vi "Set Window Icon.vi"(7 "Icon Type":enum32{"Small", "Big"}(ring), 8 "error in (no error)":errorcluster, 10 "VIRef (calling VI)":refnum<vi>, 11 "RGB Image":u32[][](array[numeric])) -> (0 "Error Out":errorcluster)   [LabVIEW 2023, in "Font Glyph Drawer Interface.lvlib" / "VI Icon Canvas.lvclass"]
doc: "Set a custom title bar icon for the referenced VI.\nIf no VI reference is supplied the VI calling this function is altered.\n\nUse <b>set</b> to change the icon to a custom icon, and <b>reset</b> to revert the icon to the previous value."
uses:
  VI Icon Canvas.lvclass
  VI Icon Canvas.lvclass/VI Icon Canvas.ctl
  user32.dll
  gdi32.dll
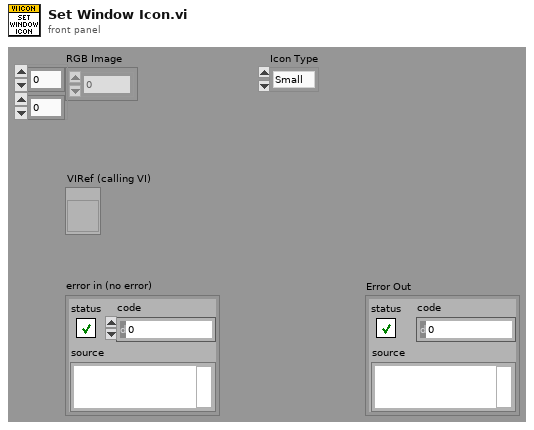
[diagram p1: front panel]
types:
  T1 = cluster{"fIcon":i32, "xHotspot":u32, "yHotspot":u32, "hbmMask":u32, "hbmColor":u32}
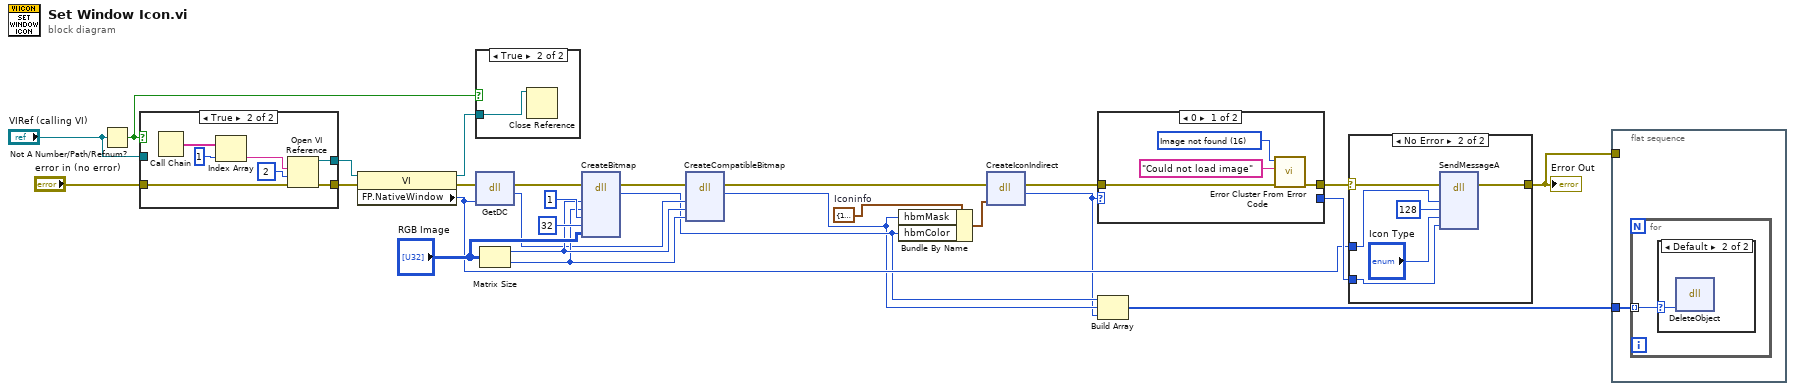
[diagram p0: block diagram]
diagram:
  w15 = T1 {"fIcon"=1, "xHotspot"=0, "yHotspot"=0, "hbmMask"=0, "hbmColor"=0}  # Iconinfo
  n1 = Not A Number/Path/Refnum?(number/path/refnum="VIRef (calling VI)") -> (NaN/Path/Refnum?=w22:bool)
  n2 = case shown="True" w22 {
    tunnel: [w29 w36] -> w26
    tunnel: "VIRef (calling VI)" -> [w29 _]
    tunnel: "error in (no error)" -> [w28 w31]
    tunnel: [w28 w30] -> w1
    frame False {
    }
    frame True {
      n3 = Call Chain() -> (call chain=w32:string[])
      n4 = Index Array(array=w32, index=1 ("Index")) -> (element=w34:string)
      n5 = Open VI Reference(vi path=w34, options=2, error in (no error)=w31) -> (vi reference=w36:refnum<vi>, error out=w30:errorcluster)  [unwired: 3 in]
    }
  }
  n6 = property class="VI"(reference=w26, error in=w1) -> (reference out=w23:refnum<vi>, error out=w12:errorcluster, "FP.NativeWindow"=w8:u64)
  n7 = case shown="True" w22 {
    tunnel: w23 -> [_ w37]
    frame False {
    }
    frame True {
      n8 = Close Reference(reference=w37) -> ()  [unwired: 1 in, 1 out]
    }
  }
  n9 = dll-call lib="user32.dll" fn="GetDC"(error in=w12, "HWND"=w8) -> (error out=w11:errorcluster, "HDC"=w13:u32)  [unwired: 3 in, 1 out]
  n10 = Matrix Size(0:"RGB Image") -> (1:w17:i32, 2:w16:i32)
  n11 = dll-call lib="gdi32.dll" fn="CreateBitmap"(error in=w11, "nWidth"=w17, "nHeight"=w16, "nPlanes"=u32 1, "nBitCount"=u32 32, "lpBits"="RGB Image") -> (error out=w18:errorcluster, "HBITMAP"=w7:u32)  [unwired: 7 in, 1 out]
  n12 = dll-call lib="gdi32.dll" fn="CreateCompatibleBitmap"(error in=w18, "hdc"=w13, "cx"=w17, "cy"=w16) -> (error out=w14:errorcluster, "HICON"=w6:u32)  [unwired: 5 in, 1 out]
  n13 = Bundle By Name(cluster=w15, "hbmMask"=w6, "hbmColor"=w7) -> (w10:T1)
  n14 = dll-call lib="user32.dll" fn="CreateIconIndirect"(error in=w14, "piconinfo"=w10) -> (error out=w9:errorcluster, "HICON"=w5:u32)  [unwired: 3 in, 1 out]
  n15 = case shown="0" w5 {
    selector: w5 -> [_ w42]
    tunnel: [_ w42] -> w24
    tunnel: [w39 w43] -> w25
    tunnel: w9 -> [w38 w43]
    frame 0 {
      w41 = 16 items=["No error", "Argument error", "Memory is full", "Out of zone", "End of file", "File already open", "Generic file I/O error", "File not found", "File permission error", "Disk is full", "Duplicate path", "Too many files open", "System feature not enabled", "Resource file not found", "Cannot add resource", "Resource not found", "Image not found", "Image memory error", "Pen does not exist", "Config type invalid", "Config token not found", "Config parse error", "Config memory error", "Bad external code format", "Bad external code offset", "External code not present", "Null window", "Destroy window error", "Null menu", "Print aborted", "Bad print record", "Print driver error", "Windows error during printing", "Memory error during printing", "Print dialog error", "Generic print error", "Invalid device refnum", "Device not found", "Device parameter error", "Device unit error", "Cannot open device", "Device call aborted", "Generic error", "Cancelled by user", "Object ID too low", "Object ID too high", "Object not in heap", "Unknown heap", "Unknown object (invalid DefProc)", "Unknown object (DefProc not in table)", "Message out of range", "Invalid (null) method", "Unknown message", "Manager call not supported", "Bad address", "Network operation in progress", "Network operation timed out", "Connection is busy", "Network attribute not supported", "Network error", "Address in use", "System out of memory", "Connection aborted", "Connection refused", "Not connected", "Already connected", "Connection closed", "Initialization error (interapplication manager)", "Bad occurrence", "Wait on unbound occurrence handler", "Occurrence queue overflow", "Datalog type conflict", "Unused", "Unrecognized type (interapplication manager)", "Memory corrupt", "Failed to make temporary DLL", "Old CIN version", "Drag socket not found", "Failed to load drop-object", "Failed to register OLE object", "Failed to release OLE object", "Format specifier type mismatch", "Unknown format specifier", "Too few format specifiers", "Too many format specifiers", "Scan failed", "Newer CIN version", "Error converting to variant", "Runtime menu error", "Password tampered", "Variant attribute not found", "Incompatible variant data type", "Event data is not available", "Event Store is not present", "Occurrence is not found", "Event Queue is not created", "Event info is not available", "Refnum passed is NULL", "Error retrieving Class GUID", "Error retrieving CoClass GUID", "Error retrieving TypeLib GUID.", "Bad built application magic bytes.", "Specific driver is different from the specific driver associated with the Logical Name.", "There is no session opened to the class driver.", "Max Error", "MAX - Error with config objects", "MAX - Error loading configuration", "MAX - Group not supported"]
      n16 = call <vilib>:"Error Cluster From Error Code.vi"("error in (no error)"=w38, "error message (\"\")"="Could not load image" ("source"), "error code (0)"=w41) -> ("error out"=w39:errorcluster)  [unwired: 6 in]
    }
    frame Default {
    }
  }
  n17 = Build Array(w7, w6, w5) -> (w4:u32[])
  n18 = case shown="No Error" w25 {
    selector: w25 -> [w44 w49]
    tunnel: [w44 w48] -> w3
    tunnel: w8 -> [_ w47]
    tunnel: w24 -> [_ w50]
    frame Error {
    }
    frame No Error {
      n19 = dll-call lib="user32.dll" fn="SendMessageA" label="SendMessage"(error in=w49, "hWnd"=w47, "uMsg"=u32 128 ("dimension size"), "wParam"="Icon Type", "lParam"=w50) -> (error out=w48:errorcluster)  [unwired: 7 in, 1 out]
    }
  }
  "Error Out" <- w3
  n20 = flat-sequence {
    tunnel: w4 -> [w51]
    tunnel: w3 -> [_]
    frame #0 {
      n21 = for {
        tunnel: w51 -> [w52] mode=indexing
        n22 = case shown="Default" w52 {
          selector: w52 -> [_ w53]
          frame 0 {
          }
          frame Default {
            n23 = dll-call lib="gdi32.dll" fn="DeleteObject"("ho"=w53) -> ()  [unwired: 5 in, 2 out]
          }
        }
      }
    }
  }
